vi "TIO Form Packet_Ser.vi"(8 "error in (no error)":errorcluster, 10 "Type":T1(ring)=enum."RPC Request", 11 "Payload":string="Q\u0017\b€dev.name") -> (0 "error out":errorcluster, 3 "Packet out":string)   [LabVIEW 2019]
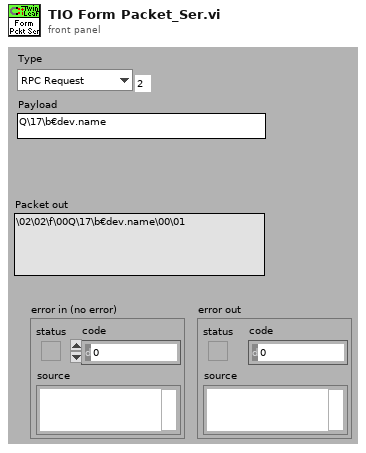
[diagram p1: front panel]
types:
  T1 = enum8{"Invalid", "Log", "RPC Request", "RPC Reply", "RPC Error", "Stream Description", "User"}
  T2 = enum16{"big-endian, network order", "native, host order", "little-endian"}
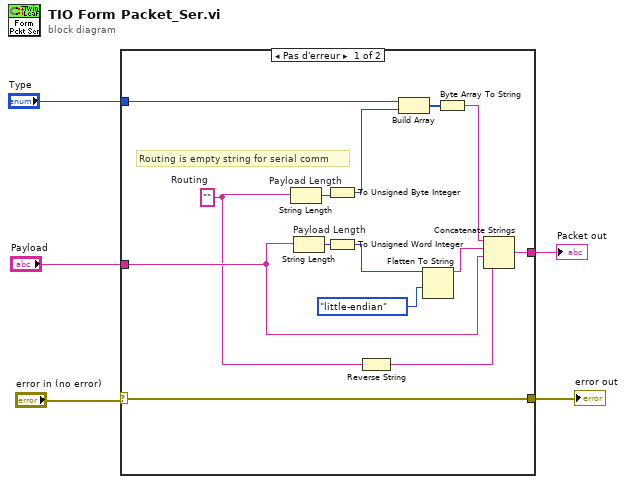
[diagram p0: block diagram]
diagram:
  n1 = case shown="Pas d'erreur" "error in (no error)" {
    selector: "error in (no error)" -> [w6 w20]
    tunnel: [w19 _] -> w5
    tunnel: "Payload" -> [w18 _]
    tunnel: "Type" -> [w13 _]
    tunnel: [w6 w20] -> w1
    frame No Error {
      w8 = ""  # Routing
      # "Routing is empty string for serial comm"
      n2 = String Length "Payload Length"(string=w8) -> (length=w12:i32)
      n3 = String Length "Payload Length"(string=w18) -> (length=w14:i32)
      n4 = To Unsigned Byte Integer(number=w12) -> (unsigned 8bit integer=w11:u8)
      n5 = To Unsigned Word Integer(number=w14) -> (unsigned 16bit integer=w16:u16)
      n6 = Reverse String(1:w8) -> (0:w7:string)
      n7 = Build Array(w13, w11) -> (w10:u8[])
      n8 = Flatten To String(anything=w16, byte order (0:big-endian, network order)=T2."little-endian") -> (data string=w15:string)  [unwired: 2 in, 2 out]
      n9 = Byte Array To String(unsigned byte array=w10) -> (string=w9:string)
      n10 = Concatenate Strings(w9, w15, w18, w7) -> (w19:string)
    }
    frame Error {
    }
  }
  "Packet out" <- w5
  "error out" <- w1
